vi "CreateKinematics.vi"() -> (3 "SWERVE_DRIVE_KINEMATICS":T1 {"SavedModuleStates"."Angle"."SIN" format="%13.4f"; "SavedModuleStates"."Angle"."COS" format="%13.4f"; "SavedModuleStates"."Angle"."VALUE" format="%13.4f"; "PrevCoR"."Y" format="%14.3f"; "PrevCoR"."X" format="%14.3f"; "Modules"."Y" format="%14.3f"; "Modules"."X" format="%14.3f"})   [LabVIEW 2023]
uses:
  <vilib>/Rock Robotics/WPI/ThirdParty/JAS_Junk/TrajLib/TypeDef/SWERVE_DRIVE_KINEMATICS.ctl
  <vilib>/Analysis/Matrix/Datatypes/RealMatrix.ctl
  <vilib>/Rock Robotics/WPI/ThirdParty/JAS_Junk/TrajLib/TypeDef/TRANSLATION2D.ctl
  <vilib>/Rock Robotics/WPI/ThirdParty/JAS_Junk/TrajLib/TypeDef/SWERVE_DRIVE_MODULE_STATE.ctl
  <vilib>/Rock Robotics/WPI/ThirdParty/JAS_Junk/TrajLib/TypeDef/ROTATION2D.ctl
  <vilib>/Rock Robotics/WPI/ThirdParty/JAS_Junk/TrajLib/Trajectory_Library.lvlib
  <vilib>/Analysis/Matrix/NI_Matrix.lvlib
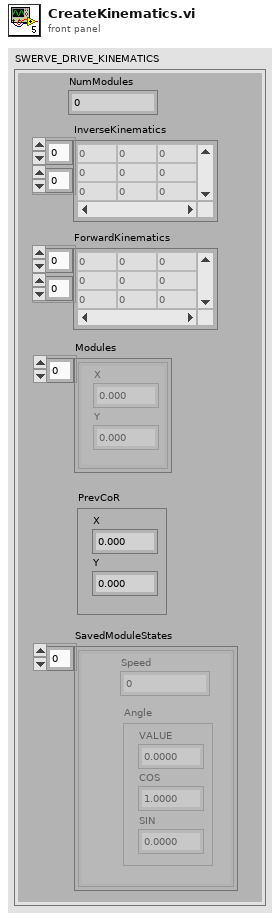
[diagram p1: front panel]
types:
  T1 = typedef "Trajectory_Library.lvlib/SWERVE_DRIVE_KINEMATICS.ctl" = cluster{"NumModules":i32, "InverseKinematics":T2, "ForwardKinematics":T2, "Modules":T3[], "PrevCoR":T3, "SavedModuleStates":T4[]}
  T2 = typedef "NI_Matrix.lvlib/RealMatrix.ctl" = dbl[][]
  T3 = typedef "Trajectory_Library.lvlib/TRANSLATION2D.ctl" = cluster{"X":dbl, "Y":dbl}
  T4 = typedef "Trajectory_Library.lvlib/SWERVE_DRIVE_MODULE_STATE.ctl" = cluster{"Speed":dbl, "Angle":T5}
  T5 = typedef "Trajectory_Library.lvlib/ROTATION2D.ctl" = cluster{"VALUE":dbl, "COS":dbl, "SIN":dbl}
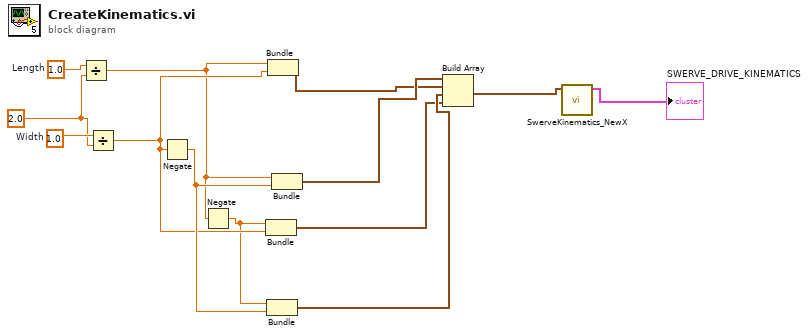
[diagram p0: block diagram]
diagram:
  w11 = 2.0 ("2")
  w12 = 1.0  # Width
  w13 = 1.0  # Length
  n1 = Divide(x=w13, y=w11) -> (x/y=w8:dbl)
  n2 = Divide(x=w12, y=w11) -> (x/y=w9:dbl)
  n3 = Negate(x=w9) -> (-x=w10:dbl)
  n4 = Negate(x=w8) -> (-x=w7:dbl)
  n5 = Bundle(w7, w9) -> (w3:cluster{dbl, dbl})  [unwired: 1 in]
  n6 = Bundle(w7, w10) -> (w4:cluster{dbl, dbl})  [unwired: 1 in]
  n7 = Bundle(w8, w9) -> (w5:cluster{dbl, dbl})  [unwired: 1 in]
  n8 = Bundle(w8, w10) -> (w6:cluster{dbl, dbl})  [unwired: 1 in]
  n9 = Build Array(w6, w5, w4, w3) -> (w1:cluster{dbl, dbl}[])
  n10 = call <vilib>:"SwerveKinematics_NewX.vi"("Wheels"=w1) -> ("SWERVE_DRIVE_KINEMATICS"=→"SWERVE_DRIVE_KINEMATICS":T1)  [unwired: 10 in]
